vi "Get Bold.vi"(8 "error in (no error)":errorcluster, 11 "Style in":refnum<class "Style.lvclass">) -> (0 "error out":errorcluster, 2 "Bold":bool, 3 "Style out":refnum<class "Style.lvclass">)   [LabVIEW 2017, in "Styles.lvlib" / "Style.lvclass"]
uses:
  Style.lvclass
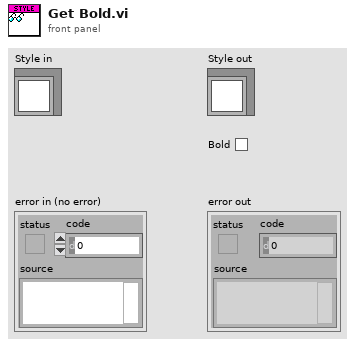
[diagram p1: front panel]
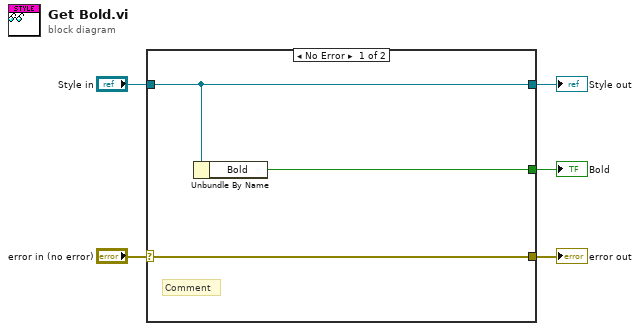
[diagram p0: block diagram]
diagram:
  n1 = case shown="No Error" "error in (no error)" {
    selector: "error in (no error)" -> [w8 w9]
    tunnel: [w8 w9] -> w4
    tunnel: [w7 w10] -> w2
    tunnel: "Style in" -> [w7 w10]
    tunnel: [w6 _] -> w1
    frame No Error {
      # "Comment"
      n2 = Unbundle By Name(w7) -> ("Bold"=w6:bool)
    }
    frame Error {
    }
  }
  "error out" <- w4
  "Style out" <- w2
  "Bold" <- w1
